vi "Adaptive Threshold (Mean).vi"(4 "Max Value (Default: 255)":u8=255, 5 "C":dbl, 6 "Invert? (Default: False)":bool, 7 "Kernel Block Size (Default: 5)":T2=enum."5", 8 "error in (no error)":errorcluster, 10 "Adaptive Threshold Result":T1, 11 "Greyscale Image-Source":T1) -> (0 "error out":errorcluster, 3 "Adaptive Threshold Result (duplicate)":T1)   [LabVIEW 2020, in "g_ar_toolkit.image.lvlib"]
uses:
  g_ar_toolkit.image.lvlib
  Kernel Block Size.ctl
  Greyscale Image.ctl
  AdaptiveThresholdMethod.ctl
  g_ar_toolkit.common/Module Path.vi
  <vilib>/Utility/error.llb/Error Cluster From Error Code.vi
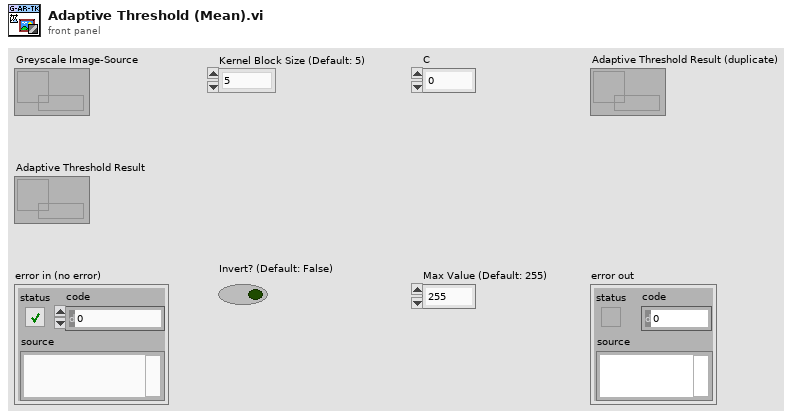
[diagram p1: front panel]
types:
  T1 = typedef "g_ar_toolkit.image.lvlib/Greyscale Image.ctl" = refnum<data-value>
  T2 = typedef "g_ar_toolkit.image.lvlib/Kernel Block Size.ctl" = enum16{"3", "5", "7", "9", "11", "13", "15", "17", "19", "21", "23", "25", "27", "29", "31", "33", "35", "37", "39", "41", "43", "45", "47", "49", "51", "53", "55", "57", "59", "61", "63", "65", "67", "69", "71", "73", "75", "77", "79", "81", "83", "85", "87", "89", "91", "93", "95", "97", "99", "101", "103", "105", "107", "109", "111", "113", "115", "117", "119", "121", "123", "125", "127", "129", "131", "133", "135", "137", "139", "141", "143", "145", "147", "149", "151", "153", "155", "157", "159", "161", "163", "165", "167", "169", "171", "173", "175", "177", "179", "181", "183", "185", "187", "189", "191", "193", "195", "197", "199", "201", "203", "205", "207", "209", "211", "213", "215", "217", "219", "221", "223", "225", "227", "229", "231", "233", "235", "237", "239", "241", "243", "245", "247", "249", "251", "253", "255", "257", "259", "261", "263", "265", "267", "269", "271", "273", "275", "277", "279", "281", "283", "285", "287", "289", "291", "293", "295", "297", "299", "301", "303", "305", "307", "309", "311", "313", "315", "317", "319", "321", "323", "325", "327", "329", "331", "333", "335", "337", "339", "341", "343", "345", "347", "349", "351", "353", "355", "357"}
  T3 = typedef "g_ar_toolkit.image.lvlib/AdaptiveThresholdMethod.ctl" = enum8{"Mean", "Gaussian"}
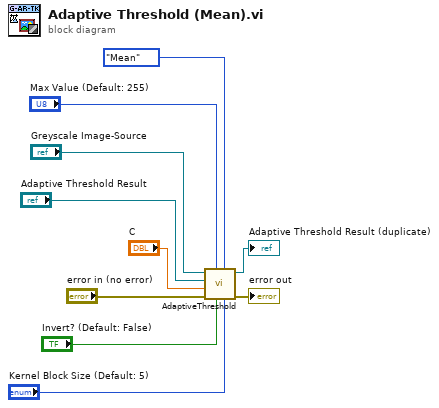
[diagram p0: block diagram]
diagram:
  n1 = call "AdaptiveThreshold.vi"("Kernel Block Size (Default: 5)"="Kernel Block Size (Default: 5)", "Adaptive Threshold Method"=AdaptiveThresholdMethod."Mean", "Invert? (Default: False)"="Invert? (Default: False)", "Max Value (Default: 255)"="Max Value (Default: 255)", "error in (no error)"="error in (no error)", "C"="C", "Adaptive Threshold Result"="Adaptive Threshold Result", "Greyscale Image-Source"="Greyscale Image-Source") -> ("error out"=→"error out":errorcluster, "Adaptive Threshold Result (duplicate)"=→"Adaptive Threshold Result (duplicate)":T1)  [unwired: 2 in]
